vi "CSMOMgr-Delete CSMO.vi"(8 "Error in":errorcluster caption="Error in (no error)", 10 "Queue Name":string, 11 "CSMOMgr":T1) -> (0 "Error out":errorcluster, 3 "CSMOMgr out":T1)   [LabVIEW 2020, in "Communicable State Machine.lvlib"]
uses:
  Communicable State Machine.lvlib
  Def-CSMOMgr.ctl
  Operation-BroadcastRegistry.ctl
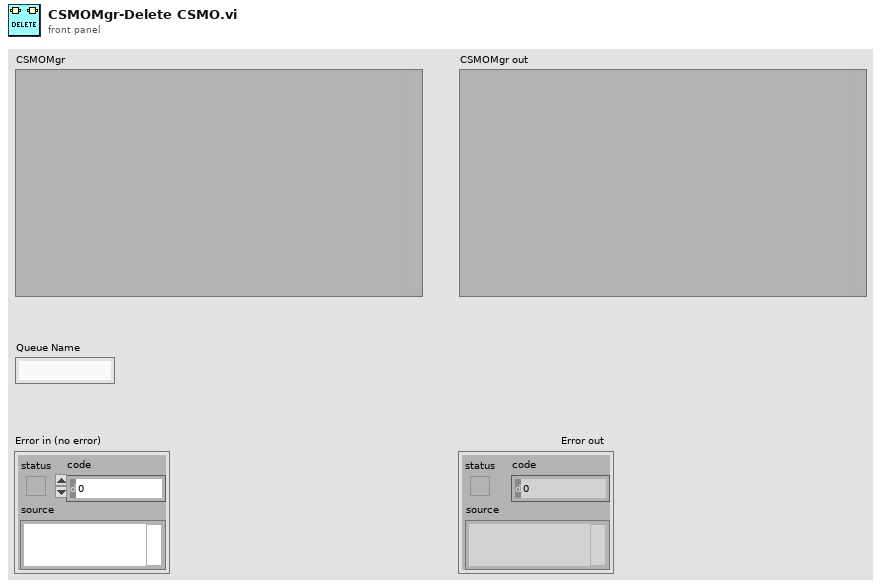
[diagram p1: front panel]
types:
  T1 = typedef "Communicable State Machine.lvlib/Def-CSMOMgr.ctl" = variant
  T2 = typedef "Communicable State Machine.lvlib/_CSMObj.ctl" = cluster{"Requested Name":string, "Module Name":string, "Mode":T3, "Queue":refnum<class "Priority Queue.lvclass">, "CSM-Data":refnum<data-value>, "User Event":refnum<user-event>, "Status Change Event":refnum<user-event>, "Allowed Messages":string[], "Mode-Data":refnum<data-value>, "Group Name":string, "Exit Event":refnum<user-event>}
  T3 = typedef "Communicable State Machine.lvlib/_CSM_MODE.ctl" = enum16{"Not Exist", "Stand Alone", "CSM", "Worker Agent", "Worker", "Chain", "Chain Node"}
  T4 = typedef "Communicable State Machine.lvlib/Operation-BroadcastRegistry.ctl" = enum16{"Delete Source Module", "Delete Target Module", "Remove Module", "Register", "Unregister", "Check", "List Status", "List Entries"}
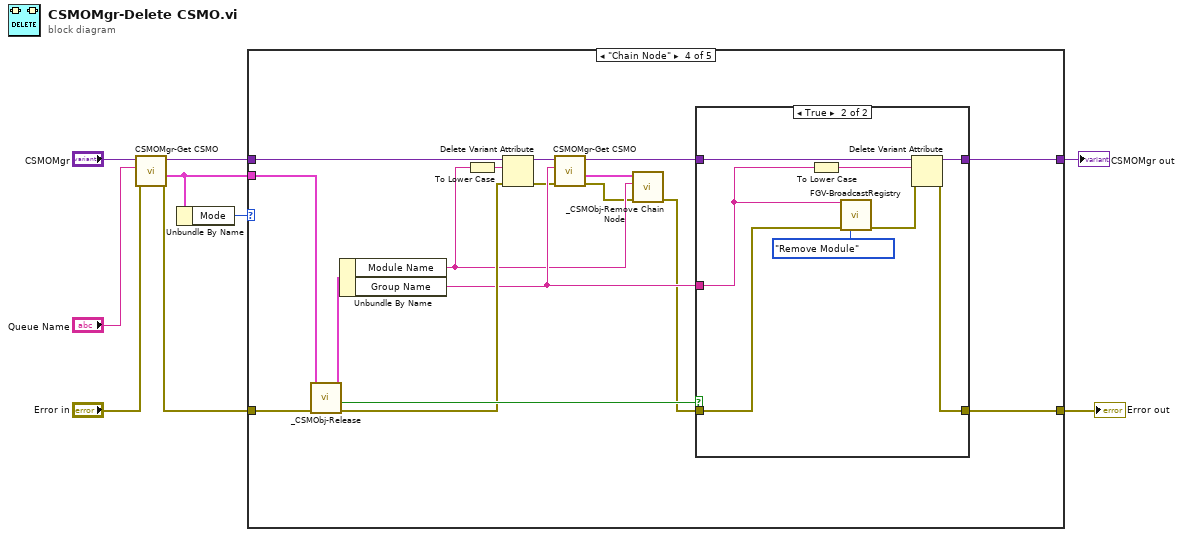
[diagram p0: block diagram]
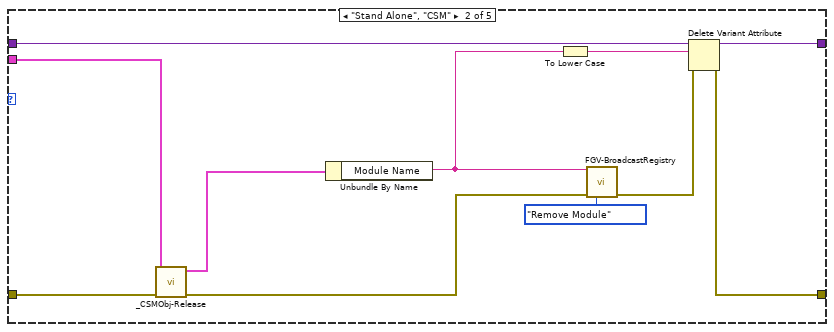
[diagram p3: hidden frame]
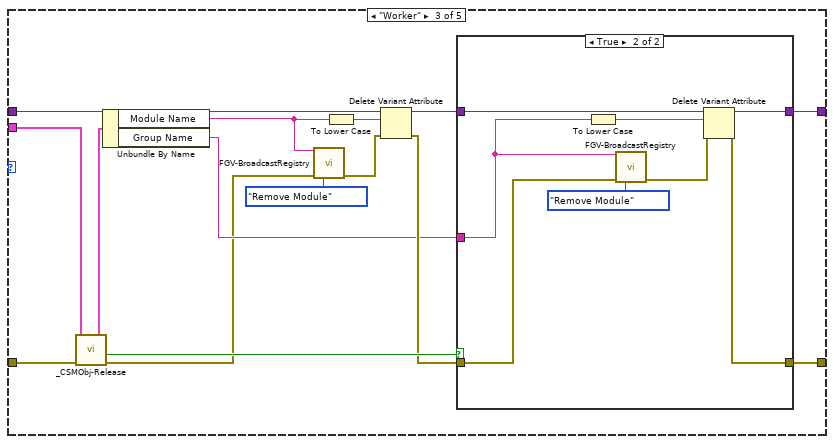
[diagram p4: hidden frame]
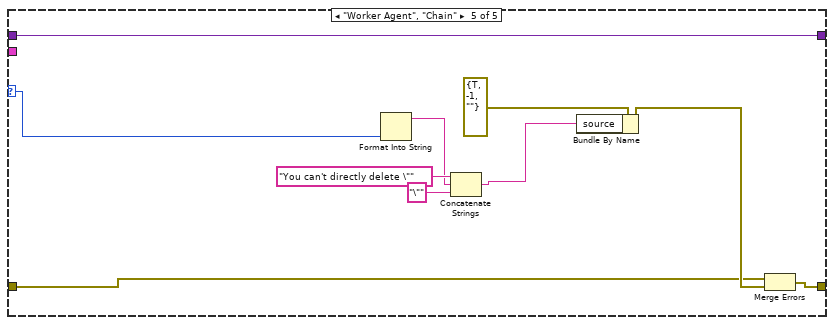
[diagram p7: hidden frame]
diagram:
  n1 = call "CSMOMgr-Get CSMO.vi"("Error in"="Error in", "Queue Name"="Queue Name", "CSMOMgr"="CSMOMgr") -> ("Error out"=w9:errorcluster, "values"=w7:T2, "CSMOMgr out"=w8:T1)  [unwired: 5 in, 1 out]
  n2 = Unbundle By Name(w7) -> ("Mode"=w6:T3)
  n3 = case shown="\"Chain Node\"" w6 {
    selector: w6 -> [_ _ _ _ w78]
    tunnel: [w11 w22 w37 w64 w84] -> w2
    tunnel: [w10 w21 w36 w63 w76] -> w1
    tunnel: w7 -> [_ w20 w35 w62 _]
    tunnel: w9 -> [w10 w19 w33 w60 w75]
    tunnel: w8 -> [w11 w18 w32 w56 w84]
    frame "Not Exist", Default {
    }
    frame "Stand Alone", "CSM" {
      n4 = call "_CSMObj-Release.vi"("Error in"=w19, "CSMQ in"=w20) -> ("Error out"=w16:errorcluster, "CSMQ out"=w17:T2)  [unwired: 7 in, 1 out]
      n5 = Unbundle By Name(w17) -> ("Module Name"=w14:string)
      n6 = To Lower Case(string=w14) -> (all lower case string=w12:string)
      n7 = call "FGV-BroadcastRegistry.vi"("Source"=w14, "Error in"=w16, "Operation"=Operation-BroadcastRegistry."Remove Module") -> ("Error out"=w15:errorcluster)  [unwired: 11 in, 1 out]
      n8 = Delete Variant Attribute(4:w15, 6:w12, 7:w18) -> (0:w21:errorcluster, 3:w22:variant)  [unwired: 1 out]
    }
    frame "Worker" {
      n9 = call "_CSMObj-Release.vi"("Error in"=w33, "CSMQ in"=w35) -> ("Error out"=w25:errorcluster, "Group Release?"=w34:bool, "CSMQ out"=w29:T2)  [unwired: 7 in]
      n10 = Unbundle By Name(w29) -> ("Module Name"=w24:string, "Group Name"=w28:string)
      n11 = call "FGV-BroadcastRegistry.vi"("Source"=w24, "Error in"=w25, "Operation"=Operation-BroadcastRegistry."Remove Module") -> ("Error out"=w26:errorcluster)  [unwired: 11 in, 1 out]
      n12 = To Lower Case(string=w24) -> (all lower case string=w23:string)
      n13 = Delete Variant Attribute(4:w26, 6:w23, 7:w32) -> (0:w30:errorcluster, 3:w31:variant)  [unwired: 1 out]
      n14 = case shown="True" w34 {
        tunnel: w28 -> [_ w44]
        tunnel: w31 -> [w39 w46]
        tunnel: [w39 w45] -> w37
        tunnel: w30 -> [w38 w43]
        tunnel: [w38 w41] -> w36
        frame False {
        }
        frame True {
          n15 = To Lower Case(string=w44) -> (all lower case string=w40:string)
          n16 = call "FGV-BroadcastRegistry.vi"("Source"=w44, "Error in"=w43, "Operation"=Operation-BroadcastRegistry."Remove Module") -> ("Error out"=w42:errorcluster)  [unwired: 11 in, 1 out]
          n17 = Delete Variant Attribute(4:w42, 6:w40, 7:w46) -> (0:w41:errorcluster, 3:w45:variant)  [unwired: 1 out]
        }
      }
    }
    frame "Chain Node" {
      n18 = call "_CSMObj-Release.vi"("Error in"=w60, "CSMQ in"=w62) -> ("Error out"=w59:errorcluster, "Group Release?"=w61:bool, "CSMQ out"=w58:T2)  [unwired: 7 in]
      n19 = Unbundle By Name(w58) -> ("Module Name"=w51:string, "Group Name"=w57:string)
      n20 = To Lower Case(string=w51) -> (all lower case string=w48:string)
      n21 = Delete Variant Attribute(4:w59, 6:w48, 7:w56) -> (0:w53:errorcluster, 3:w55:variant)  [unwired: 1 out]
      n22 = call "CSMOMgr-Get CSMO.vi"("Error in"=w53, "Queue Name"=w57, "CSMOMgr"=w55) -> ("Error out"=w50:errorcluster, "values"=w52:T2, "CSMOMgr out"=w54:T1)  [unwired: 5 in, 1 out]
      n23 = call "_CSMObj-Remove Chain Node.vi"("Error in"=w50, "Requested Name"=w51, "CSMObj in"=w52) -> ("Error out"=w49:errorcluster)  [unwired: 7 in, 1 out]
      n24 = case shown="True" w61 {
        tunnel: w57 -> [_ w71]
        tunnel: w54 -> [w66 w73]
        tunnel: [w66 w72] -> w64
        tunnel: w49 -> [w65 w70]
        tunnel: [w65 w68] -> w63
        frame False {
        }
        frame True {
          n25 = To Lower Case(string=w71) -> (all lower case string=w67:string)
          n26 = call "FGV-BroadcastRegistry.vi"("Source"=w71, "Error in"=w70, "Operation"=Operation-BroadcastRegistry."Remove Module") -> ("Error out"=w69:errorcluster)  [unwired: 11 in, 1 out]
          n27 = Delete Variant Attribute(4:w69, 6:w67, 7:w73) -> (0:w68:errorcluster, 3:w72:variant)  [unwired: 1 out]
        }
      }
    }
    frame "Worker Agent", "Chain" {
      n28 = Format Into String(w78) -> (resulting string=w80:string)  [unwired: 3 in, 1 out]
      n29 = Concatenate Strings("You can't directly delete \"" ("source"), w80, "\"" ("source")) -> (w79:string)
      n30 = Bundle By Name(cluster=errorcluster {"status"=TRUE, "code"=-1, "source"=""} ("error out"), "source"=w79) -> (w77:errorcluster)
      n31 = Merge Errors(w75, w77) -> (w76:errorcluster)
    }
  }
  "Error out" <- w1
  "CSMOMgr out" <- w2
